vi "Do.vi"(8 "error in (no error)":errorcluster, 10 "Actor in":refnum<class "Actor.lvclass">, 11 "Update Channel Data Msg in":refnum<class "Update Channel Data Msg.lvclass">) -> (0 "error out":errorcluster, 2 "Actor out":refnum<class "Actor.lvclass">)   [LabVIEW 2015, in "Sequencer.lvlib" / "Update Channel Data Msg.lvclass"]
doc: "(<B>Filename</B>: Actor Framework.lvlib:Message.lvclass:Do.vi)\n\nDefines what a message does when it is received by an actor. Generally, a message instructs an actor to invoke one of its methods. By default, this method does nothing. A child class must override it to define behavior. Create a child class by using the Actor Framework Message Maker dialog box."
uses:
  Update Channel Data Msg.lvclass
  <vilib>/ActorFramework/Actor/Actor.lvclass
  Sequencer/Sequencer.lvclass
  Update Channel Data Msg.lvclass/Update Channel Data Msg.ctl
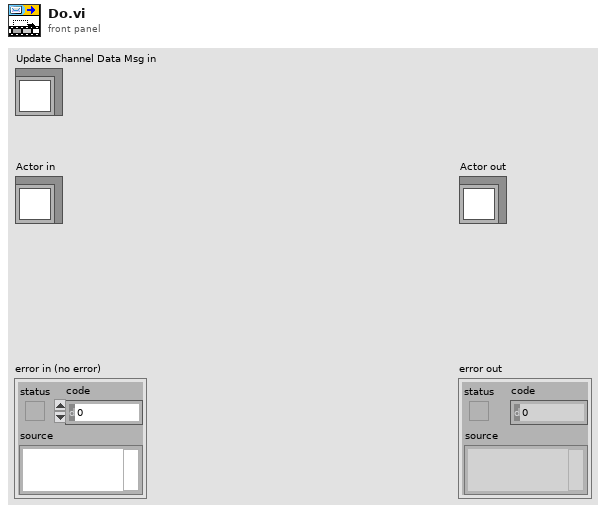
[diagram p1: front panel]
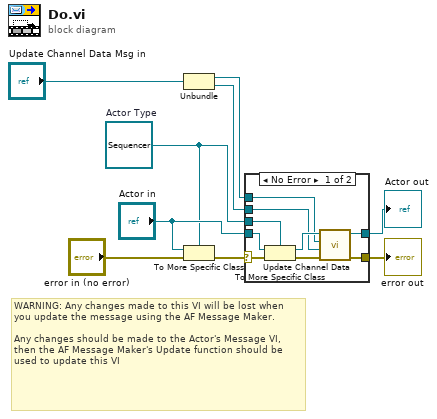
[diagram p0: block diagram]
diagram:
  w4 = refnum<class "Sequencer.lvclass"> refnum  # Actor Type
  # "WARNING: Any changes made to this VI will be lost when you update the message using the AF Message Maker.\n\nAny changes should be made to the Actor's Message VI, then the AF Message Maker's Update function should be used to update this VI"
  n1 = Unbundle("Update Channel Data Msg in") -> (w3:refnum<class "Message Enqueuer.lvclass">, w2:refnum<class "ChannelData.lvclass">)
  n2 = To More Specific Class(target class=w4, reference="Actor in", error in="error in (no error)") -> (error out=w8:errorcluster)  [unwired: 1 out]
  n3 = case shown="No Error" w8 {
    selector: w8 -> [w18 w20]
    tunnel: [w13 w20] -> w7
    tunnel: [w12 w19] -> w6
    tunnel: "Actor in" -> [w17 w19]
    tunnel: w4 -> [w16 _]
    tunnel: w3 -> [w11 _]
    tunnel: w2 -> [w10 _]
    frame No Error {
      n4 = To More Specific Class ("Actor Cast")(target class=w16, reference=w17, error in=w18) -> (specific class reference=w15:refnum<class "Sequencer.lvclass">, error out=w14:errorcluster)
      n5 = call "Update Channel Data.vi"("Sequencer in"=w15, "Channel Enququer"=w11, "ChannelData"=w10, "error in (no error)"=w14) -> ("Sequencer out"=w12:refnum<class "Sequencer.lvclass">, "error out"=w13:errorcluster)  [unwired: 5 in]
    }
    frame Error {
    }
  }
  "error out" <- w7
  "Actor out" <- w6
